vi "AIDI-Read (DI).vi"(0 "Task In":refnum<k21>, 7 "number of samples per channel":i32=-1, 11 "error in (no error)":errorcluster) -> (4 "Task Out":refnum<k21>, 8 "DO Waveforms":bool[][](array[boolean]), 15 "error out":errorcluster)   [LabVIEW 2020]
uses:
  <vilib>/DAQmx/read.llb/DAQmx Read (Digital Wfm 1Chan NSamp).vi
  <vilib>/DAQmx/miscellaneous.llb/DAQmx Fill In Error Info.vi
  <vilib>/Waveform/DWDTOps.llb/DWDT Digital to Boolean Array.vi
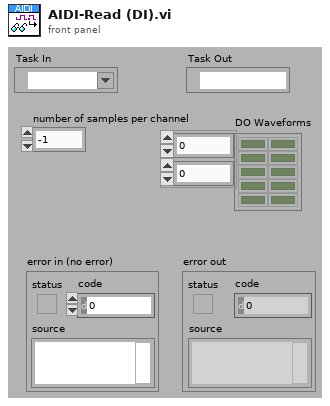
[diagram p1: front panel]
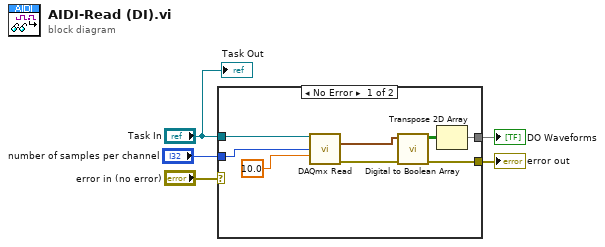
[diagram p0: block diagram]
diagram:
  n1 = case shown="No Error" "error in (no error)" {
    selector: "error in (no error)" -> [_ w14]
    tunnel: [w9 w14] -> w5
    tunnel: "Task In" -> [w13 _]
    tunnel: [w6 _] -> w2
    tunnel: "number of samples per channel" -> [w8 _]
    frame No Error {
      n2 = call-poly <vilib>:"DAQmx Read.vi"("task/channels in"=w13, "number of samples per channel"=w8, "timeout"=10.0) -> ("data"=w11:digitalwaveform, "error out"=w12:errorcluster)  [unwired: 10 in, 1 out]
      n3 = call-poly <vilib>:"Digital to Boolean Array.vi"("error in (no error)"=w12, "digital waveform"=w11) -> ("error out"=w9:errorcluster, "boolean array"=w10:bool[][])  [unwired: 8 in]
      n4 = Transpose 2D Array(2D array=w10) -> (transposed array=w6:bool[][])
    }
    frame Error {
    }
  }
  "error out" <- w5
  "DO Waveforms" <- w2
  "Task Out" <- "Task In"
